vi "Open.vi"(8 "error in (no error)":errorcluster, 11 "VISA resource name":refnum<visa-resource-name>) -> (0 "error out":errorcluster, 3 "VISA Refnum out":refnum<visa-resource-name>)   [LabVIEW 2019, in "RP100.lvlib"]
uses:
  RP100.lvlib
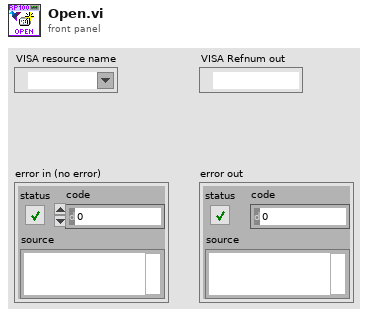
[diagram p1: front panel]
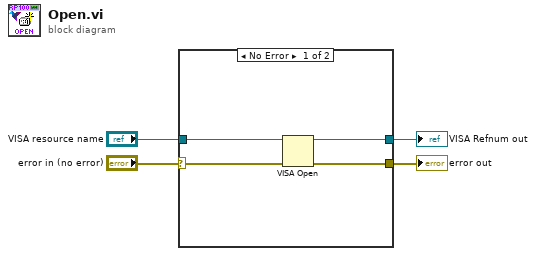
[diagram p0: block diagram]
diagram:
  n1 = case shown="No Error" "error in (no error)" {
    selector: "error in (no error)" -> [w7 w10]
    tunnel: [w5 w9] -> w4
    tunnel: "VISA resource name" -> [w8 w9]
    tunnel: [w6 w10] -> w2
    frame No Error {
      n2 = VISA Open(error in (no error)=w7, VISA resource name=w8) -> (VISA resource name=w5:refnum<visa-resource-name>, error out=w6:errorcluster)  [unwired: 3 in]
    }
    frame Error {
    }
  }
  "VISA Refnum out" <- w4
  "error out" <- w2
